vi "STAGE+mono+counter_edit15.vi"() -> ()   [LabVIEW 2017]
panel:
  out "XY Graph 2":cluster{dbl[], dbl[]}[](graph)
  out "XY Graph":cluster{dbl[], dbl[]}(graph)
  out "PROGRESS":u8(slide) max=10 step=10 scale=0.0..5.0
  in  "?":enum32{"DELAY", "COUNTER", "MONO", "PLOT"}(tab)
  out "Final time [ps]":dbl
  out "Current time [ps]":dbl
  out "Initial time [ps]":dbl
  in  "Set this as t0":bool
  in  "Axis":i32=1
  in  "Motor ON":bool
  in  "Motor OFF":bool
  out "Current Position [mm]":dbl
  out "Final Position [mm]":dbl
  in  "Data Points":i32=100
  out "Current Point":i32
  in  "Step Size [um]":i32=10
  in  "Target [mm]":dbl format="%.3f"
  in  "Move":bool
  out "Initial position [mm]":dbl
  in  "GPIB address":string="23"
  in  "Count Mode":u16(ring) items=["A,B for Preset T", "A-B for Preset T", "A+B for Preset T", "A for Preset B"]
  in  "Trigger mode":u16(ring) items=["10 MHz"=0, "Input 2"=2, "Input T"=3]
  in  "Channel A Input":u16(ring)=1 items=["10 MHz", "Input 1"]
  in  "Channel B Input":u16(ring)=2 items=["Input 1"=1, "Input 2"=2]
  in  "Number of Measurements\n to take at one point/ Number of Periods":u16=1 min=1 max=2000 step=1
  in  "Time between measurements\n at one point (s)/Dwell Time":dbl=0.002 min=0.002 max=60.0 step=0.001
  in  "gate A mode (CW:0)":i16(slide) scale=0.0..2.0 scale format="%.2f"
  out "Counts":i32
  in  "Integrating time \nin 10^-7 sec":dbl=10000000.0
  out "Grating #":dbl
  out "Blaze angle":dbl
  out "Grooves/mm":dbl
  out "Mono port":T1(ring)
  out "Time delay":u32=450000 min=1
  in  "Step size":dbl=10.0 min=0.0
  in  "Scan to":i32=4000
  in  "Scan from":i32=2600
  out "Current wavelength":dbl
  in  "?":bool
  in  "Array":dbl[](array[numeric])
  out "Numeric":i32
  out "Numeric 2":i32
  out "Timeout 2":bool
  in  "?":bool
  out "Timeout":bool
  in  "Collect Data!":bool
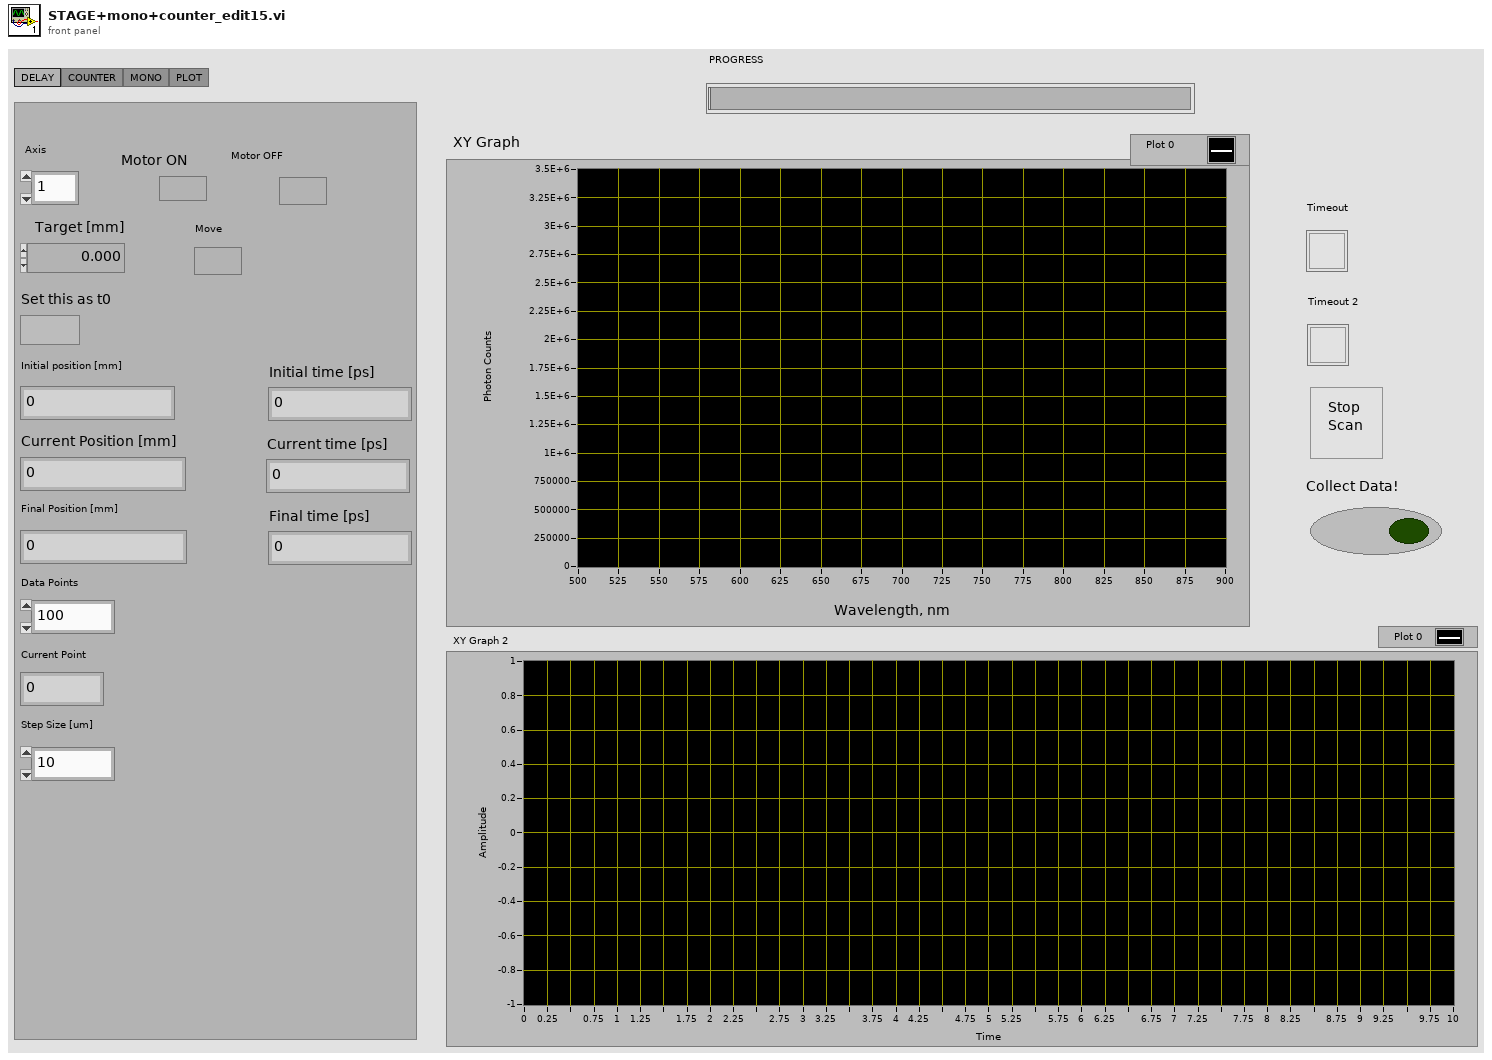
[diagram p1: front panel]
types:
  T1 = enum8{"COM 1", "COM 2", "COM 3", "COM 4", "COM 5", "COM 6", "COM 7", "COM 8", "COM 9"}
  T2 = cluster{"input XON/XOFF":bool, "input HW Handshake":bool, "input alt HW HShk":bool, "output XON/XOFF":bool, "output HW Handshake":bool, "output alt HW HShk":bool, "XOFF byte":u8, "XON byte":u8, "parity error byte":u16}
  T3 = enum16{"no parity", "odd parity", "even parity", "mark parity", "space parity"}
  T4 = cluster{"Y[0]":dbl, "Y[1]":dbl, "Y[2]":dbl, "Y[3]":dbl, "Y[4]":dbl, "Y[5]":dbl, "Y[6]":dbl, "Y[7]":dbl, "Y[8]":dbl}
  T5 = typedef "NI_Matrix.lvlib/RealMatrix.ctl" = dbl[][]
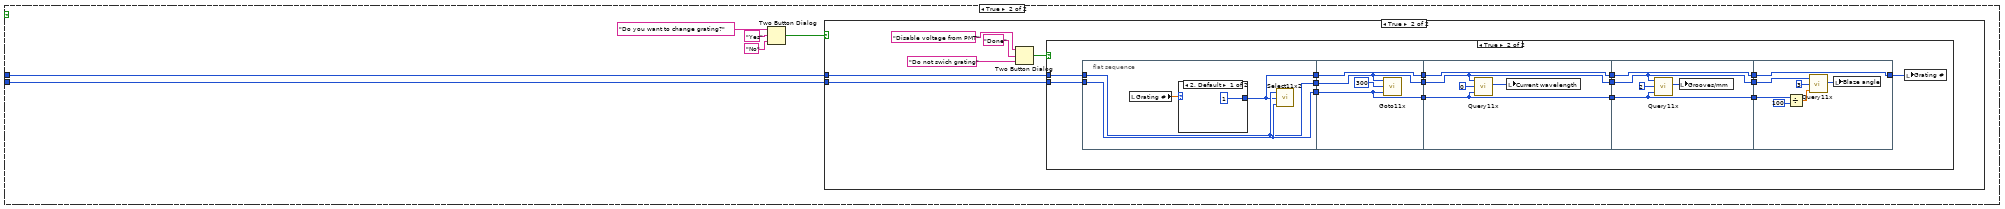
[diagram p2: hidden frame]
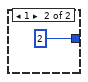
[diagram p5: hidden frame]
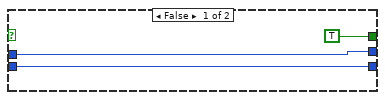
[diagram p6: hidden frame]
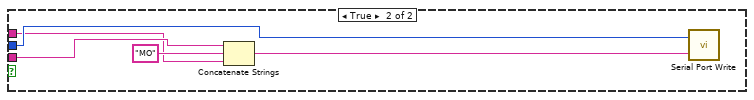
[diagram p7: hidden frame]
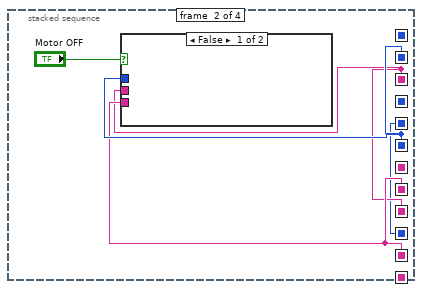
[diagram p8: hidden frame]
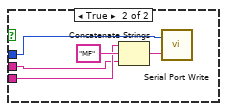
[diagram p9: hidden frame]
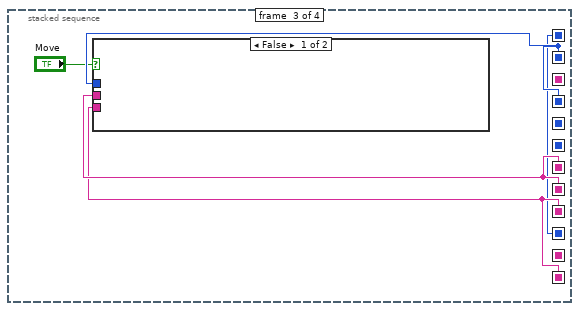
[diagram p10: hidden frame]
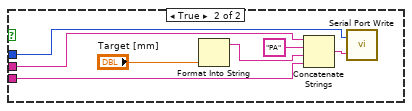
[diagram p11: hidden frame]
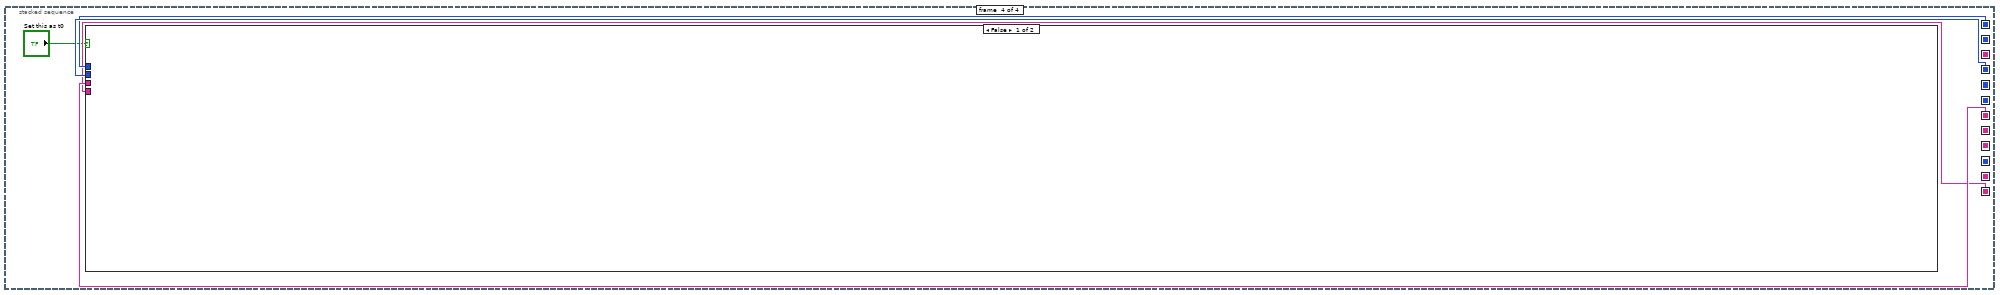
[diagram p12: hidden frame]
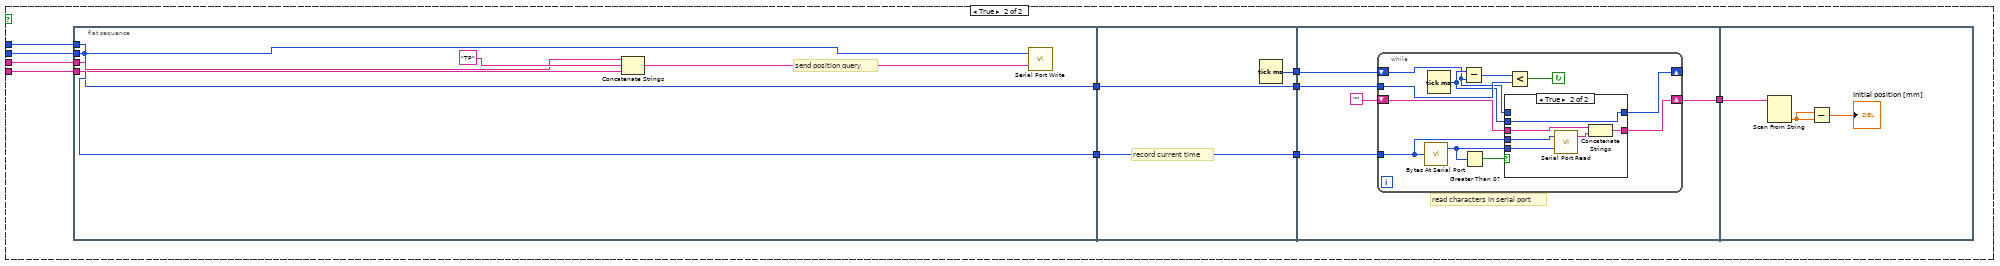
[diagram p13: hidden frame]
diagram:
  (unwired) FALSE
  w39 = u32 19200  # baud rate
  w38 = u16 8  # data bits
  w37 = enum16{"1 bit", "1.5 bits", "2 bits"}."1 bit"  # stop bits
  w41 = T3."no parity"  # parity
  w36 = 4  # 0=COM1 so n=COM(n+1)
  w40 = u16 1024  # buffer size
  n1 = flat-sequence {
    tunnel: ["Data Points"] -> w45
    tunnel: "Axis" -> [w67]
    tunnel: [w59] -> w44
    tunnel: [w67] -> w43
    tunnel: ["Step Size [um]"] -> w17
    tunnel: [w59] -> w16
    tunnel: ["Step Size [um]"] -> w15
    tunnel: ["Data Points"] -> w14
    tunnel: [w59] -> w13
    tunnel: [w58] -> w12
    tunnel: [w59] -> w10
    tunnel: [w58] -> w9
    tunnel: [w61] -> w8
    tunnel: [w51] -> w7
    tunnel: w45 -> [w151]
    tunnel: w44 -> [w150]
    tunnel: w43 -> [w149]
    tunnel: w36 -> [w145]
    tunnel: "GPIB address" -> [w144]
    tunnel: "GPIB address" -> [w143]
    tunnel: w17 -> [w131]
    tunnel: w16 -> [w129]
    tunnel: w15 -> [w128]
    tunnel: w14 -> [w126]
    tunnel: w13 -> [w121]
    tunnel: w12 -> [w120]
    tunnel: "Integrating time \nin 10^-7 sec" -> [w119]
    tunnel: w10 -> [w117]
    tunnel: w9 -> [w116]
    tunnel: w8 -> [w115]
    tunnel: w7 -> [w113]
    tunnel: w3 -> [w94]
    tunnel: w2 -> [w93]
    tunnel: w1 -> [w92]
    frame #0 {
      n2 = while {
        stop <- "Collect Data!" stop-if-true
        n3 = Multiply(x=1, y=1000) -> (x*y=w49:i32)
        n4 = Wait (ms)(milliseconds to wait=w49) -> ()  [unwired: 1 out]
      }
    }
    frame #1 {
      w52 = 1000000000000.0
      w57 = 1000
      w60 = 300000000
      w62 = 1000
      n5 = local read "Initial position [mm]"() -> (w59:dbl)
      n6 = Multiply(x="Step Size [um]", y="Data Points") -> (x*y=w66:i32)
      n7 = Divide(x=w66, y=w62) -> (x/y=w65:dbl)
      n8 = Divide(x="Step Size [um]", y=w62) -> (x/y=w61:dbl)
      n9 = Add(x=w59, y=w65) -> (x+y=w58:dbl)
      "Final Position [mm]" <- w58
      n10 = Divide(x=w59, y=w57) -> (x/y=w55:dbl)
      n11 = Divide(x=w58, y=w57) -> (x/y=w56:dbl)
      n12 = Divide(x=w55, y=w60) -> (x/y=w54:dbl)
      n13 = Divide(x=w56, y=w60) -> (x/y=w53:dbl)
      n14 = Multiply(x=w53, y=w52) -> (x*y=→"Final time [ps]":dbl)
      n15 = Multiply(x=w54, y=w52) -> (x*y=w51:dbl)
      "Initial time [ps]" <- w51
    }
    frame #2 {
      w74 = "\r\n"
      n16 = Increment(x=w126) -> (x+1=w127:i32)
      n17 = Divide(x=w131, y=1000.0) -> (x/y=w107:dbl)
      n18 = for {
        N: w127 -> [_]
        tunnel: w107 -> [w162]
        tunnel: w129 -> [w160]
        tunnel: [w153] -> w125 mode=indexing
        i -> [w161]
        # "distances"
        n19 = Multiply(x=w162, y=w161) -> (x*y=w159:dbl)
        n20 = Add(x=w160, y=w159) -> (x+y=w158:dbl)
        n21 = Divide(x=w158, y=1000) -> (x/y=w152:dbl)
        n22 = Divide(x=w152, y=300000000) -> (x/y=w155:dbl)
        n23 = Multiply(x=w155, y=1000000000000.0) -> (x*y=w153:dbl)
      }
      n24 = Multiply(x="Scan to", y=1) -> (x*y=w114:i32)
      n25 = Multiply(x=1, y="Scan from") -> (x*y=w103:i32)
      n26 = Divide(x=w107, y=1000.0) -> (x/y=w108:dbl)
      n27 = Subtract(x=w114, y=w103) -> (x-y=w138:i32)
      n28 = local read "Numeric 2"() -> (w96:i32)
      n29 = local read "Numeric"() -> (w95:i32)
      n30 = Divide(x=w138, y="Step size") -> (x/y=w137:dbl)
      n31 = Divide(x=w108, y=300000000) -> (x/y=w110:dbl)
      n32 = Multiply(x=w110, y=1000000000000.0) -> (x*y=w106:dbl)
      n33 = Build Array(w113) -> (w100:dbl[])
      n34 = Round Toward -Infinity(1:w137) -> (0:w136:dbl)
      n35 = Concatenate Strings("\r", "\n") -> (w146:string)
      n36 = Initialize Array(0, w95, w96) -> (w98:i32[][])
      n37 = Increment(x=w136) -> (x+1=w102:dbl)
      n38 = for {
        N: w151 -> [w213]
        tunnel: w150 -> [w240]
        tunnel: w128 -> [w236]
        tunnel: w149 -> [w233]
        tunnel: w146 -> [w230]
        tunnel: w145 -> [w231]
        tunnel: w144 -> [w229]
        tunnel: w93 -> [w226]
        tunnel: w94 -> [w228]
        tunnel: w143 -> [w227]
        tunnel: [w178] -> w134 mode=indexing
        tunnel: w103 -> [w221]
        tunnel: "Step size" -> [w220]
        tunnel: w136 -> [w219]
        tunnel: w121 -> [_]
        tunnel: w120 -> [_]
        tunnel: w119 -> [w218]
        tunnel: "Scan to" -> [w217]
        tunnel: "Scan from" -> [w216]
        tunnel: "Step size" -> [w187]
        tunnel: w117 -> [w208]
        tunnel: w116 -> [w206]
        tunnel: w115 -> [w209]
        tunnel: w106 -> [w196]
        shift-right: [w180] -> _
        shift-left: w100 -> [w190]
        shift-right: [w179] -> _
        shift-left: dbl[] [] ("Y") -> [w185]
        tunnel: w113 -> [w214]
        tunnel: "Scan from" -> [w188]
        tunnel: "Step size" -> [w189]
        shift-right: [w177] -> _
        shift-left: w100 -> [w183]
        shift-right: [w175] -> _
        shift-left: w98 -> [w174]
        tunnel: w94 -> [w170]
        tunnel: w93 -> [w169]
        tunnel: w92 -> [w168]
        i -> [w195]
        w207 = 1000
        w210 = 300000000
        n39 = To Time Stamp(1:w221) -> ()  [unwired: 1 out]
        n40 = property on="PROGRESS" class="Slide (strict)"("Scale.Increment"=1, "Scale.Maximum"=w213, "Scale.Minimum"=0) -> ()  [unwired: 2 in, 2 out]
        n41 = stacked-sequence {
          tunnel: w226 -> [w412]
          tunnel: w227 -> [_]
          frame #0 {
            n42 = call <vilib>:"Close Serial Driver.vi"("port number"=w412) -> ()  [unwired: 1 out]
            n43 = GPIB Misc(0:"loc 23" ("command string")) -> ()  [unwired: 1 in, 3 out]
          }
        }
        n44 = Multiply(x=w196, y=w195) -> (x*y=w215:dbl)
        n45 = Divide(x=w208, y=w207) -> (x/y=w204:dbl)
        n46 = Divide(x=w206, y=w207) -> (x/y=w203:dbl)
        n47 = Divide(x=w209, y=w207) -> (x/y=w205:dbl)
        n48 = Number To Decimal String(number=w218) -> (decimal integer string=w224:string)  [unwired: 1 in]
        n49 = Build Array(w188) -> (w192:i32[])
        n50 = Add(x=1, y=w195) -> (x+y=→"PROGRESS":i32)
        n51 = Divide(x=w236, y=1000) -> (x/y=w235:dbl)
        n52 = Divide(x=w204, y=w210) -> (x/y=w198:dbl)
        n53 = Divide(x=w203, y=w210) -> (x/y=w197:dbl)
        n54 = Divide(x=w205, y=w210) -> (x/y=w199:dbl)
        n55 = Add(x=w214, y=w215) -> (x+y=w184:dbl)
        n56 = Concatenate Strings("CP 2,", w224) -> (w222:string)
        n57 = flat-sequence {
          tunnel: w229 -> [w257]
          tunnel: w228 -> [w256]
          tunnel: w226 -> [w255]
          tunnel: w221 -> [w254]
          tunnel: w220 -> [w253]
          tunnel: w219 -> [w252]
          tunnel: w217 -> [w251]
          tunnel: w216 -> [w250]
          tunnel: w192 -> [w249]
          tunnel: dbl[] [] ("Y") -> [w248]
          tunnel: w189 -> [w247]
          tunnel: w188 -> [w246]
          tunnel: w187 -> [w245]
          tunnel: [w244] -> w186
          tunnel: w170 -> [w243]
          tunnel: w169 -> [w242]
          tunnel: w168 -> [w241]
          tunnel: w186 -> [w366]
          tunnel: w185 -> [w373]
          tunnel: [w366] -> w182
          tunnel: w181 -> [w370]
          tunnel: [w368] -> w180
          tunnel: [w367] -> w179
          tunnel: [w366] -> w178
          tunnel: w182 -> [w382]
          tunnel: [w375] -> w177
          tunnel: w176 -> [w376]
          tunnel: w174 -> [w379]
          tunnel: [w377] -> w175
          frame #0 {
            # "step size"
            n58 = while {
              tunnel: w255 -> [_]
              tunnel: w256 -> [_]
              tunnel: w257 -> [w290]
              tunnel: w254 -> [w289]
              tunnel: w253 -> [w288]
              tunnel: w252 -> [w287]
              tunnel: w251 -> [w272]
              tunnel: w250 -> [w273]
              tunnel: w245 -> [w274]
              tunnel: w247 -> [w285]
              shift-right: [w281] -> w244
              shift-left: w248 -> [w280]
              shift-right: [w275] -> _
              shift-left: w249 -> [w283]
              tunnel: w246 -> [w278]
              tunnel: w243 -> [w261]
              tunnel: w242 -> [w260]
              tunnel: w241 -> [w259]
              i -> [w286]
              stop <- w293 stop-if-true
              n59 = property on="XY Graph" class="XYGraph (strict)"("XScale.Increment"=w274, "XScale.Maximum"=w272, "XScale.Minimum"=w273) -> ()  [unwired: 2 in, 2 out]
              n60 = Multiply(x=w286, y=w288) -> (x*y=w294:dbl)
              n61 = Multiply(x=w286, y=w285) -> (x*y=w284:dbl)
              n62 = Greater Or Equal?(x=w286, y=w287) -> (x >= y?=w291:bool)
              n63 = Add(x=w284, y=w278) -> ()  [unwired: 1 out]
              n64 = Add(x=w294, y=w289) -> (x+y=w258:dbl)
              n65 = Or(x="?", y=w291) -> (x .or. y?=w293:bool)
              n66 = flat-sequence {
                tunnel: w290 -> [w309]
                tunnel: w258 -> [w310]
                tunnel: [w310] -> w265
                tunnel: [w296] -> w264
                tunnel: [w295] -> w263
                tunnel: [w309] -> w262
                tunnel: w261 -> [w299]
                tunnel: w260 -> [w298]
                tunnel: w259 -> [w297]
                tunnel: [w343] -> w271
                tunnel: [w342] -> w270
                tunnel: [w340] -> w269
                tunnel: w265 -> [w344]
                tunnel: w264 -> [w343]
                tunnel: w263 -> [w342]
                tunnel: w262 -> [w340]
                tunnel: w271 -> [w351]
                tunnel: w270 -> [w350]
                tunnel: w269 -> [w345]
                tunnel: [w345] -> w268
                tunnel: w268 -> [w353]
                tunnel: [w353] -> w267
                tunnel: w267 -> [w354]
                tunnel: [w354] -> w266
                tunnel: [w360] -> w277
                tunnel: w266 -> [w361]
                frame #0 {
                  n67 = flat-sequence {
                    tunnel: w299 -> [w316]
                    tunnel: [w316] -> w308
                    tunnel: w298 -> [w318]
                    tunnel: [w318] -> w307
                    tunnel: w297 -> [w314]
                    tunnel: [w314] -> w306
                    tunnel: w308 -> [w322]
                    tunnel: [w322] -> w305
                    tunnel: w307 -> [w323]
                    tunnel: [w323] -> w304
                    tunnel: w306 -> [w320]
                    tunnel: [w320] -> w303
                    tunnel: w305 -> [w331]
                    tunnel: [w331] -> w302
                    tunnel: w304 -> [w328]
                    tunnel: [w328] -> w301
                    tunnel: w303 -> [w326]
                    tunnel: [w326] -> w300
                    tunnel: w302 -> [w333]
                    tunnel: w301 -> [w334]
                    tunnel: w300 -> [_]
                    tunnel: [w334] -> w296
                    tunnel: [w333] -> w295
                    frame #0 {
                      n68 = call "Query11x.vi"("port number"=w318, "QUERY"=u16 0, "time delay"=w316) -> ("timeout"=w315:bool, "STATUS MESSAGE"=w313:u16)  [unwired: 2 out]
                      n69 = local write "Timeout"(w315) -> ()
                      n70 = Divide(x=w313, y=1 ("Numeric")) -> (x/y=→"Current wavelength":dbl)
                    }
                    frame #1 {
                      n71 = call "Query11x.vi"("port number"=w323, "QUERY"=u16 2, "time delay"=w322) -> ("timeout"=w321:bool, "STATUS MESSAGE"=→"Grooves/mm":u16)  [unwired: 2 out]
                      n72 = local write "Timeout"(w321) -> ()
                    }
                    frame #2 {
                      n73 = Divide(x=w331, y=i16 100 ("device (1)")) -> (x/y=w329:dbl)
                      n74 = call "Query11x.vi"("port number"=w328, "QUERY"=u16 3, "time delay"=w329) -> ("timeout"=w327:bool, "STATUS MESSAGE"=→"Blaze angle":u16)  [unwired: 2 out]
                      n75 = local write "Timeout"(w327) -> ()
                    }
                    frame #3 {
                      n76 = Divide(x=w333, y=i16 100 ("device (1)")) -> (x/y=w337:dbl)
                      n77 = call "Query11x.vi"("port number"=w334, "QUERY"=u16 4, "time delay"=w337) -> ("timeout"=w336:bool, "STATUS MESSAGE"=→"Grating #":u16)  [unwired: 2 out]
                      n78 = local write "Timeout"(w336) -> ()
                    }
                  }
                }
                frame #1 {
                  n79 = call "Goto11x.vi"("time delay"=w342, "WAVELENGTH"=w344, "port number"=w343) -> ("timeout"=w341:bool)  [unwired: 2 out]
                  n80 = local write "Timeout 2"(w341) -> ()
                }
                frame #2 {
                  # "set counter time in 10^-7 seconds in CW"
                  n81 = call "Query11x.vi"("port number"=w351, "QUERY"=0, "time delay"=w350) -> ("timeout"=w349:bool, "STATUS MESSAGE"=w348:u16)  [unwired: 2 out]
                  n82 = local write "Timeout 2"(w349) -> ()
                  n83 = Divide(x=w348, y=1) -> (x/y=w347:dbl)
                  n84 = local write "Current wavelength"(w347) -> ()
                }
                frame #3 {
                  n85 = call "Start.vi"("GPIB Address"=w353) -> ()  [unwired: 9 in]
                }
                frame #4 {
                  # "Wait for Scan to Finish"
                  n86 = for {
                    N: 1 -> [_]
                    tunnel: w354 -> [w356]
                    n87 = while {
                      tunnel: w356 -> [w357]
                      stop <- w359 stop-if-true
                      n88 = call "ScanDone.vi"("Wait (ms)"=1000, "GPIB Address"=w357) -> ("Scan Finished?"=w359:bool)
                    }
                  }
                }
                frame #5 {
                  n89 = call "Read Data.vi"("Channel Number"=0, "GPIB Address"=w361, "Number of Datapoints"=1) -> ("Data"=w362:i32[])
                  n90 = Index Array(array=w362, index=0) -> (element=w360:i32)
                  "Counts" <- w360
                }
              }
              n91 = Build Array (concatenate)(w283, w258) -> (w282:dbl[])
              n92 = Build Array (concatenate)(w280, w277) -> (w279:dbl[])
              n93 = Bundle(w282, w279) -> (w276:cluster{dbl[], dbl[]})  [unwired: 1 in]
              "XY Graph" <- w276
              n94 = Unbundle(w276) -> (w275:dbl[], w281:dbl[])
            }
          }
          frame #1 {
            n95 = Array To Cluster(array=w366) -> (cluster=w374:T4)
            n96 = Unbundle By Name(w374) -> ("Y[5]"=w372:dbl)  [unwired: 10 out]
            n97 = Build Array (concatenate)(w373, w372) -> (w371:dbl[])
            n98 = Bundle(w370, w371) -> (w369:cluster{dbl[], dbl[]})  [unwired: 1 in]
            n99 = Unbundle(w369) -> (w368:dbl[], w367:dbl[])
          }
          frame #2 {
            n100 = Array Size(array="Array") -> (size(s)=w380:i32)
            n101 = flat-sequence {
              tunnel: w382 -> [w387]
              tunnel: "Array" -> [w386]
              tunnel: w380 -> [w385]
              tunnel: [w383] -> w378
              tunnel: w379 -> [w404]
              tunnel: w378 -> [w403]
              tunnel: [w401] -> w377
              tunnel: w376 -> [w400]
              tunnel: [w399] -> w375
              frame #0 {
                n102 = for {
                  N: w385 -> [w389]
                  tunnel: w386 -> [w397]
                  tunnel: w387 -> [w391]
                  tunnel: [w388] -> w384
                  i -> [w396]
                  n103 = local read "Scan from"() -> (w394:i32)
                  n104 = Index Array(array=w397, index=w396) -> (element=w395:dbl)
                  n105 = local read "Step size"() -> (w392:dbl)
                  n106 = Subtract(x=w395, y=w394) -> (x-y=w393:dbl)
                  n107 = Divide(x=w393, y=w392) -> (x/y=w390:dbl)
                  n108 = Index Array(array=w391, index=w390) -> (element=w388:dbl)
                  "Numeric" <- w389
                }
                n109 = Build Array(w384) -> (w383:dbl[])
              }
              frame #1 {
                n110 = local read "Numeric"() -> (w402:i32)
                n111 = Build Array (concatenate)(w404, w403) -> (w401:dbl[][])
                n112 = for {
                  N: w402 -> [_]
                  tunnel: w401 -> [w410]
                  tunnel: w400 -> [w408]
                  tunnel: [w407] -> w399
                  tunnel: [w405] -> w398 mode=indexing
                  i -> [w409]
                  n113 = Index Array(array=w410, index (row)=w409) -> (element=w406:dbl[])  [unwired: 1 in]
                  n114 = Bundle(w408, w406) -> (w405:cluster{dbl[], dbl[]})  [unwired: 1 in]
                  n115 = Unbundle(w405) -> (w407:dbl[])  [unwired: 1 out]
                }
                "XY Graph 2" <- w398
              }
            }
          }
        }
        n116 = Multiply(x=w235, y=w195) -> (x*y=w239:dbl)
        n117 = Multiply(x=w198, y=1000000000000.0) -> (x*y=w172:dbl)
        n118 = Multiply(x=w197, y=1000000000000.0) -> (x*y=w171:dbl)
        n119 = Multiply(x=w199, y=1000000000000.0) -> (x*y=w173:dbl)
        n120 = Build Array (concatenate)(w190, w184) -> (w181:dbl[])
        n121 = Build Array (concatenate)(w183, w184) -> (w176:dbl[])
        n122 = property on="XY Graph 2" class="XYGraph (strict)"("XScale.Increment"=w173, "XScale.Maximum"=w171, "XScale.Minimum"=w172) -> ()  [unwired: 2 in, 2 out]
        n123 = Add(x=w240, y=w239) -> (x+y=w238:dbl)
        n124 = Format Into String(w233) -> (resulting string=w232:string)  [unwired: 3 in, 1 out]
        n125 = GPIB Write(0:w229, 1:w222, 2:i16 5 ("mode (0)")) -> ()  [unwired: 2 in, 2 out]
        n126 = flat-sequence {
          tunnel: w238 -> [w415]
          tunnel: [w415] -> w234
          tunnel: w230 -> [w417]
          tunnel: w232 -> [w416]
          tunnel: w231 -> [w413]
          tunnel: w234 -> [w426]
          frame #0 {
            n127 = Format Into String(w415) -> (resulting string=w414:string)  [unwired: 3 in, 1 out]
            n128 = Wait (ms)(milliseconds to wait=u32 100) -> ()  [unwired: 1 out]
            n129 = Concatenate Strings(w416, "PA" ("Substring"), w414, w417) -> (w419:string)
            n130 = call <vilib>:"Serial Port Write.vi"("string to write"=w419, "port number"=w413) -> ()  [unwired: 1 out]
          }
          frame #1 {
            n131 = Divide(x=w426, y=1000) -> (x/y=w424:dbl)
            n132 = Wait (ms)(milliseconds to wait=u32 1000) -> ()  [unwired: 1 out]
            n133 = Divide(x=w424, y=300000000) -> (x/y=w423:dbl)
            n134 = Multiply(x=w423, y=1000000000000.0) -> (x*y=→"Current time [ps]":dbl)
            "Current Position [mm]" <- w426
          }
        }
        "Current Point" <- w195
        "Numeric 2" <- w213
      }
      n135 = for {
        N: w102 -> [_]
        tunnel: "Step size" -> [w167]
        tunnel: w103 -> [w165]
        tunnel: [w163] -> w101 mode=indexing
        i -> [w166]
        # "wavelengths"
        n136 = Multiply(x=w167, y=w166) -> (x*y=w164:dbl)
        n137 = Add(x=w165, y=w164) -> (x+y=w163:dbl)
      }
      n138 = Build Array (concatenate)(0, w125) -> (w68:dbl[])
      n139 = Build Array(w101) -> (w135:dbl[][])
      n140 = local read "Integrating time \nin 10^-7 sec"() -> (w72:dbl)
      n141 = Transpose Matrix(1:w134) -> (0:w132:dbl[][])
      n142 = Transpose Matrix(1:w135) -> (0:w133:dbl[][])
      n143 = Build Array (concatenate)(w133, w132) -> (w69:T5)
      n144 = Insert Into Array(array=w69, index (row)=0, new element=w68) -> (w122:T5)  [unwired: 1 in]
      n145 = local read "Blaze angle"() -> (w91:dbl)
      n146 = local read "Grating #"() -> (w90:dbl)
      n147 = Multiply(x=w72, y=1e-07) -> (x*y=w71:dbl)
      n148 = Get Date/Time In Seconds() -> (seconds since 1Jan1904=w84:timestamp)
      n149 = Array To Spreadsheet String(delimiter (Tab)=",", array=w122, 3:"%f" ("format string")) -> (spreadsheet string=w73:string)
      n150 = Number To Decimal String(number=w91) -> (decimal integer string=w75:string)  [unwired: 1 in]
      n151 = Format Date/Time String(time format string (%c)="%Y-%b-%d %H:%M:%S", seconds (now)=w84) -> (date/time string=w85:string)  [unwired: 1 in]
      n152 = Number To Decimal String(number=w71) -> (decimal integer string=w86:string)  [unwired: 1 in]
      n153 = Number To Decimal String(number=w90) -> (decimal integer string=w87:string)  [unwired: 1 in]
      n154 = call <vilib>:"Space Constant.vi"() -> ("String"=w88:string)
      n155 = Concatenate Strings(w74, "Data was taken on ", w85, w74, "Integration Time is ", w86, w88, "s", w74, "Monochromator gratng # ", w87, "; ", "blazed for ", w75, w88, "nm", w74, w74, w74, w73) -> (w89:string)
      n156 = Write to Text File(text=w89) -> ()  [unwired: 3 in, 3 out]
    }
  }
  n157 = flat-sequence {
    tunnel: [w430] -> w30
    tunnel: [w429] -> w29
    frame #0 {
      n158 = call "CM Com Read ini.vi"() -> ("Mono port"=w429:T1, "time delay1"=w430:u32)  [unwired: 7 in]
    }
  }
  n159 = call <vilib>:"Serial Port Init.vi"("flow control etc."=T2 {"input XON/XOFF"=FALSE, "input HW Handshake"=FALSE, "input alt HW HShk"=FALSE, "output XON/XOFF"=FALSE, "output HW Handshake"=FALSE, "output alt HW HShk"=FALSE, "XOFF byte"=13, "XON byte"=11, "parity error byte"=0}, "parity"=w41, "buffer size"=w40, "stop bits"=w37, "data bits"=w38, "baud rate"=w39, "port number"=w36) -> ("error code"=w35:i32)
  n160 = call "CM Serial Port Setup.vi"("COM port"=w29, "time delay"=w30) -> ("time delay1"=w25:u32, "DK port Out"=w26:T1, "error code"=w28:i32)  [unwired: 7 in]
  n161 = Equal To 0?(x=w28) -> (x = 0?=w27:bool)
  n162 = Concatenate Strings("\r", "\n") -> (w31:string)
  n163 = while {
    tunnel: w36 -> [w433]
    tunnel: w31 -> [w434]
    tunnel: w35 -> [_]
    tunnel: "Axis" -> [w431]
    stop <- TRUE continue-if-true
    w432 = u32 200  # timeout
    n164 = Format Into String(w431) -> (resulting string=w435:string)  [unwired: 3 in, 1 out]
    n165 = stacked-sequence {
      seq-local: [w440 _ _ _] -> [_ w451 _ _]
      seq-local: [w439 _ _ _] -> [_ w450 _ _]
      seq-local: [w441 _ _ _] -> [_ w452 _ _]
      seq-local: [w438 _ _ _] -> [_ w448 _ _]
      seq-local: [_ w451 _ _] -> [_ _ w461 _]
      seq-local: [_ w450 _ _] -> [_ _ w460 _]
      seq-local: [_ w452 _ _] -> [_ _ w462 _]
      seq-local: [_ w448 _ _] -> [_ _ w458 _]
      seq-local: [_ _ w461 _] -> [_ _ _ w474]
      seq-local: [_ _ w460 _] -> [_ _ _ w471]
      seq-local: [_ _ w462 _] -> [_ _ _ w473]
      seq-local: [_ _ w458 _] -> [_ _ _ w472]
      tunnel: w435 -> [w440 _ _ _]
      tunnel: w434 -> [w439 _ _ _]
      tunnel: w433 -> [w441 _ _ _]
      tunnel: w432 -> [w438 _ _ _]
      frame #0 {
        n166 = case shown="False" "Motor ON" {
          tunnel: w441 -> [_ w447]
          tunnel: w440 -> [_ w444]
          tunnel: w439 -> [_ w443]
          frame False {
          }
          frame True {
            n167 = Concatenate Strings(w444, "MO" ("Substring"), w443) -> (w445:string)
            n168 = call <vilib>:"Serial Port Write.vi"("string to write"=w445, "port number"=w447) -> ()  [unwired: 1 out]
          }
        }
      }
      frame #1 {
        n169 = case shown="False" "Motor OFF" {
          tunnel: w452 -> [_ w457]
          tunnel: w451 -> [_ w454]
          tunnel: w450 -> [_ w453]
          frame False {
          }
          frame True {
            n170 = Concatenate Strings(w454, "MF" ("Substring"), w453) -> (w455:string)
            n171 = call <vilib>:"Serial Port Write.vi"("string to write"=w455, "port number"=w457) -> ()  [unwired: 1 out]
          }
        }
      }
      frame #2 {
        n172 = case shown="False" "Move" {
          tunnel: w462 -> [_ w469]
          tunnel: w461 -> [_ w466]
          tunnel: w460 -> [_ w465]
          frame False {
          }
          frame True {
            n173 = Format Into String("Target [mm]") -> (resulting string=w463:string)  [unwired: 3 in, 1 out]
            n174 = Concatenate Strings(w466, "PA" ("Substring"), w463, w465) -> (w467:string)
            n175 = call <vilib>:"Serial Port Write.vi"("string to write"=w467, "port number"=w469) -> ()  [unwired: 1 out]
          }
        }
      }
      frame #3 {
        n176 = case shown="False" "Set this as t0" {
          tunnel: w474 -> [_ w484]
          tunnel: w473 -> [_ w483]
          tunnel: w472 -> [_ w482]
          tunnel: w471 -> [_ w481]
          frame False {
          }
          frame True {
            n177 = flat-sequence {
              tunnel: w484 -> [w488]
              tunnel: w483 -> [w487]
              tunnel: [w487] -> w480
              tunnel: w482 -> [w485]
              tunnel: [w485] -> w479
              tunnel: w481 -> [w486]
              tunnel: w480 -> [w492]
              tunnel: [w492] -> w478
              tunnel: w479 -> [w491]
              tunnel: [w491] -> w477
              tunnel: [w493] -> w476
              tunnel: w478 -> [w498]
              tunnel: w477 -> [w496]
              tunnel: w476 -> [w495]
              tunnel: [w494] -> w475
              tunnel: w475 -> [w520]
              frame #0 {
                # "send position query"
                n178 = Concatenate Strings(w488, "TP" ("Substring"), w486) -> (w489:string)
                n179 = call <vilib>:"Serial Port Write.vi"("string to write"=w489, "port number"=w487) -> ()  [unwired: 1 out]
              }
              frame #1 {
                # "record current time"
                n180 = Tick Count (ms)() -> (millisecond timer value=w493:u32)
              }
              frame #2 {
                # "read characters in serial port"
                n181 = while {
                  shift-left: w495 -> [w499]
                  shift-right: [w500] -> _
                  tunnel: w496 -> [w503]
                  shift-left: "" -> [w506]
                  shift-right: [w505] -> w494
                  tunnel: w498 -> [w507]
                  stop <- w502 continue-if-true
                  n182 = call <vilib>:"Bytes At Serial Port.vi"("port number"=w507) -> ("byte count"=w508:u32)  [unwired: 1 out]
                  n183 = Tick Count (ms)() -> (millisecond timer value=w501:u32)
                  n184 = Subtract(x=w501, y=w499) -> (x-y=w504:u32)
                  n185 = Greater Than 0?(x=w508) -> (x > 0?=w509:bool)
                  n186 = case shown="True" w509 {
                    tunnel: w508 -> [_ w517]
                    tunnel: w507 -> [_ w516]
                    tunnel: w506 -> [w511 w514]
                    tunnel: [w511 w513] -> w505
                    tunnel: [w510 w512] -> w500
                    tunnel: w501 -> [_ w512]
                    tunnel: w499 -> [w510 _]
                    frame False {
                    }
                    frame True {
                      n187 = call <vilib>:"Serial Port Read.vi"("requested byte count"=w517, "port number"=w516) -> ("string read"=w515:string)  [unwired: 1 out]
                      n188 = Concatenate Strings(w514, w515) -> (w513:string)
                    }
                  }
                  n189 = Less?(x=w504, y=w503) -> (x < y?=w502:bool)
                }
              }
              frame #3 {
                n190 = Scan From String(input string=w520) -> (output 1=w518:dbl)  [unwired: 4 in, 3 out]
                n191 = Subtract(x=w518, y=w518) -> (x-y=→"Initial position [mm]":dbl)
              }
            }
          }
        }
      }
    }
    n192 = Wait Until Next ms Multiple(millisecond multiple=u32 50) -> ()  [unwired: 1 out]
  }
  n193 = case shown="True" w27 {
    tunnel: w26 -> [w523 w526]
    tunnel: w25 -> [w522 w525]
    tunnel: [w523 w526] -> w2
    tunnel: [w522 w525] -> w3
    tunnel: [TRUE FALSE] -> w1
    frame False {
    }
    frame True {
      n194 = call "CM Com Write ini.vi"("time delay1"=w526, "Mono port"=w525) -> ()  [unwired: 7 in]
      n195 = local write "Mono port"(w526) -> ()
      n196 = local write "Time delay"(w525) -> ()
    }
  }
  n197 = case shown="False" "?" {
    tunnel: w3 -> [_ w528]
    tunnel: w2 -> [_ w527]
    frame False {
    }
    frame True {
      n198 = Two Button Dialog(message="Do you want to change grating?", 1:"No" ("F button name (\"Cancel\")"), 2:"Yes" ("T button name (\"OK\")")) -> (T button?=w529:bool)
      n199 = case shown="True" w529 {
        tunnel: w528 -> [_ w534]
        tunnel: w527 -> [_ w533]
        frame False {
        }
        frame True {
          n200 = Two Button Dialog(message="Disable voltage from PMT", 1:"Do not swich grating" ("F button name (\"Cancel\")"), 2:"Done" ("T button name (\"OK\")")) -> (T button?=w535:bool)
          n201 = case shown="True" w535 {
            tunnel: w534 -> [_ w553]
            tunnel: w533 -> [_ w552]
            frame False {
            }
            frame True {
              n202 = flat-sequence {
                tunnel: w553 -> [w557]
                tunnel: [w557] -> w550
                tunnel: w552 -> [w556]
                tunnel: [w556] -> w549
                tunnel: [w554] -> w548
                tunnel: w550 -> [w561]
                tunnel: [w561] -> w547
                tunnel: w549 -> [w562]
                tunnel: [w562] -> w546
                tunnel: w548 -> [w560]
                tunnel: [w560] -> w545
                tunnel: w547 -> [w568]
                tunnel: [w568] -> w544
                tunnel: w546 -> [w567]
                tunnel: [w567] -> w543
                tunnel: w545 -> [w565]
                tunnel: [w565] -> w542
                tunnel: w544 -> [w571]
                tunnel: [w571] -> w541
                tunnel: w543 -> [w572]
                tunnel: [w572] -> w540
                tunnel: w542 -> [w570]
                tunnel: [w570] -> w539
                tunnel: w541 -> [w576]
                tunnel: w540 -> [w577]
                tunnel: [w575] -> w551
                tunnel: w539 -> [w575]
                frame #0 {
                  n203 = local read "Grating #"() -> (w555:dbl)
                  n204 = case shown="2, Default" w555 {
                    tunnel: [1 2] -> w554
                    frame 2, Default {
                    }
                    frame 1 {
                    }
                  }
                  n205 = call "Select11x2.vi"("time delay"=w557, "NEW GRT?"=w554, "port number"=w556) -> ()  [unwired: 3 out]
                }
                frame #1 {
                  n206 = call "Goto11x.vi"("time delay"=w561, "WAVELENGTH"=u16 300, "port number"=w562) -> ()  [unwired: 3 out]
                }
                frame #2 {
                  n207 = call "Query11x.vi"("port number"=w567, "QUERY"=u16 0, "time delay"=w568) -> ("STATUS MESSAGE"=w564:u16)  [unwired: 3 out]
                  n208 = local write "Current wavelength"(w564) -> ()
                }
                frame #3 {
                  n209 = call "Query11x.vi"("port number"=w572, "QUERY"=u16 2, "time delay"=w571) -> ("STATUS MESSAGE"=w569:u16)  [unwired: 3 out]
                  n210 = local write "Grooves/mm"(w569) -> ()
                }
                frame #4 {
                  n211 = Divide(x=w576, y=i16 100 ("device (1)")) -> (x/y=w578:dbl)
                  n212 = call "Query11x.vi"("port number"=w577, "QUERY"=u16 3, "time delay"=w578) -> ("STATUS MESSAGE"=w574:u16)  [unwired: 3 out]
                  n213 = local write "Blaze angle"(w574) -> ()
                }
              }
              n214 = local write "Grating #"(w551) -> ()
            }
          }
        }
      }
    }
  }
  n215 = call "Configure.vi"("Dwell Time (s)"="Time between measurements\n at one point (s)/Dwell Time", "Channel T Input"="Trigger mode", "Channel B Input"="Channel B Input", "Channel A Input"="Channel A Input", "Integrating time, 10^-7 sec"="Integrating time \nin 10^-7 sec", "gate mode (CW:0)"="gate A mode (CW:0)", "Scan End Mode"=FALSE, "Number of Periods"="Number of Measurements\n to take at one point/ Number of Periods", "Count Mode"="Count Mode", "GPIB Address"="GPIB address") -> ()
  "Mono port" <- w29
  "Time delay" <- w30
